vi "RealTimeSingleOld_NotInUse.vi"(4 "Frames/s":sgl=2.0, 5 "return to start":bool, 6 "Scan Axis":i8=3, 7 "Motion Board ID":T4=1 min=1 max=32 step=1, 8 "BKPT Shift":i32=75, 9 "stop":bool) -> (0 "error out":errorcluster, 2 "Bd ID Out":T3)   [LabVIEW 2022 SP3]
uses:
  ScanningControl/Motion Controllers/-MotionRoutines/MotionGlobals.vi
  <instrlib>/Acqiris Dx/Acqiris Dx.lvlib
  <vilib>/Motion/FlexMotion/FunctionsVIs/Trajectory.llb/Load Acceleration/Deceleration.flx
  <vilib>/Motion/FlexMotion/CustomControls/CustomControls.llb/Axis To Control.flx
  <vilib>/Motion/FlexMotion/CustomControls/CustomControls.llb/Program.flx
  <instrlib>/Newport ESP301/Newport ESP301.lvlib
  <instrlib>/niScope/Acquire/Fetch/niScope Multi Fetch Binary 8.vi
  ScanningControl/-ScanSystem/DataHandling/ReverseDataI8.vi
  <vilib>/DAQmx/write.llb/DAQmx Write (Digital 1D Bool NChan 1Samp 1Line).vi
  <instrlib>/LeCroy Wave Series/LeCroy Wave Series.lvlib
  <vilib>/Motion/FlexMotion/FunctionsVIs/Trajectory.llb/Wait for Move Complete (8 axes).flx
  <vilib>/Motion/FlexMotion/FunctionsVIs/StartStopMotion.llb/Start Motion (8 axes).flx
  <vilib>/Motion/FlexMotion/FunctionsVIs/StartStopMotion.llb/Stop Motion (8 axes).flx
panel:
  in  "Filter Prams":T1={"low cutoff"=20, "order"=81, "high cutoff"=60}
  in  "Type of Mean":u16(ring) items=["Mean from lines", "Mean just lines", "Poly Mean", "No mean", "Filter"]
  in  "Stop Motor":bool
  in  "Axis Tune":enum32{"Axis 1", "Axis 2", "Axis 3", "Axis 4"}(radio)=enum."Axis 2"
  in  "Position (mm) (Abs)":dbl format="%.3f"
  in  "Tabor":T2={"Time Step (ms)"=5000, "Burst Ct"=[1, 3, 5, 10, 20], "Voltage Steps"=[100.0], "Tabor Step Through?"=FALSE} {"Voltage Steps" format="%_3g"}
  in  "*.eye":bool
  in  "Movie Name":string="none"
  in  "BMP?":bool
  in  "view":bool=TRUE
  in  "distance?":bool=TRUE
  in  "Display mode":u16(ring)=1 items=["Linear Abs Grey", "Log Grey Scale", "Linear Color Scale", "Sector"]
  out "Raw data":dbl[][](graph)
  out "Frames":i32
  # "Cross Axis Motion"
  # "Set for 8 bit data"
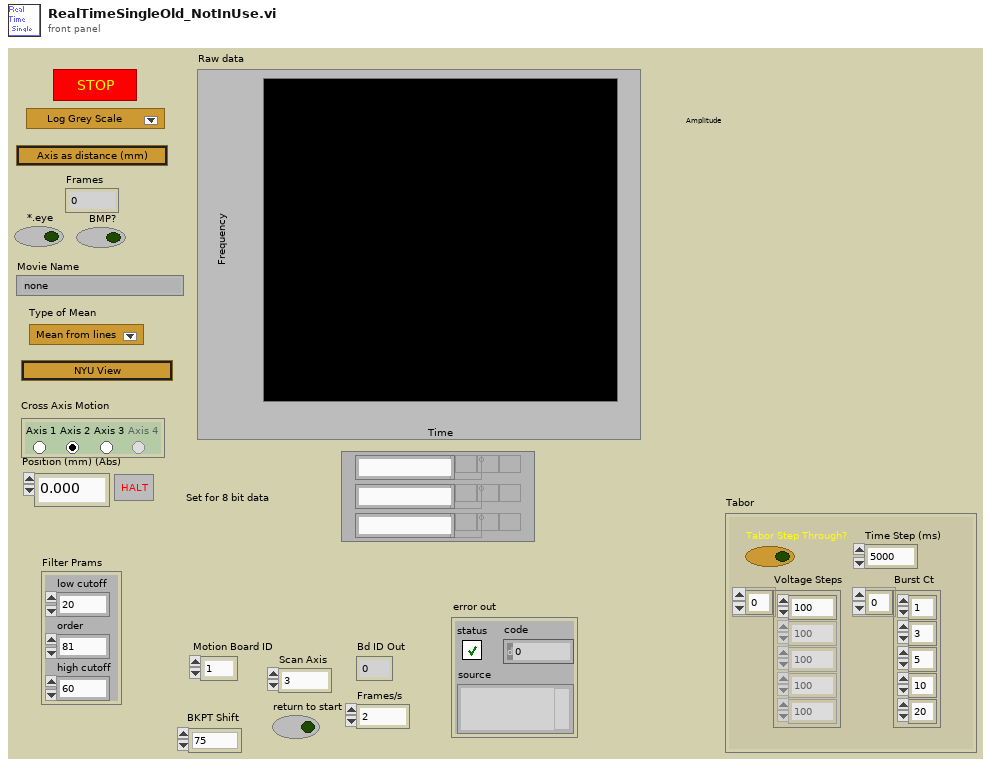
[diagram p1: front panel]
types:
  T1 = cluster{"low cutoff":i32, "order":i32, "high cutoff":i32}
  T2 = cluster{"Time Step (ms)":i64, "Burst Ct":i8[], "Voltage Steps":sgl[], "Tabor Step Through?":bool}
  T3 = typedef "Bd Id Out" = u8
  T4 = typedef "Board Id" = u8
  T5 = typedef "location.ctl" = enum16{"Automatic", "WCM Main", "Hawaii", "Columbia MM3000", "Columbia  NI System", "NYU", "RRI 2", "UHI Allen", "CUMC RT", "Chiba", "Stony Brook", "WCM Microscopy", "WCM Aeoretch", "WCM Optics Lab", "WCM Main 2Axis", "WCM Rotation", "WCM SAM SMAC", "SERI GP"}
  T6 = typedef "Program.flx" = u8
  T7 = cluster{"delay":sgl, "pivot distance":sgl, "sector scan angle":sgl, "operator":string, "Scan Mode":string, "location":string}
  T8 = cluster{"gain":dbl, bool, "Array":i16[][], "gain 2":dbl}
  T9 = typedef "Resource Out (Enum).flx" = u16
  T10 = typedef "Axis To Control.flx" = u16
  T11 = cluster{"X right":dbl, "X left":dbl, "Y low":dbl, "Y high":dbl}
  T12 = cluster{"Axis scaling Params":cluster{"X right":dbl, "X left":dbl, "Y low":dbl, "Y high":dbl}, "x scaled":dbl[][], "y scaled":dbl[][], "scales":cluster{"inc x (mm)":dbl, "inc y (mm)":dbl}, dbl[][]}
  T13 = cluster{"returnedSamplesPerSeg":i32, "indexFirstPoint":i32, "sampTime":dbl, "vGain":dbl, "vOffset":dbl, "returnedSegments":i32, "nbrAvgWforms":i32, "actualTriggersInAcqLo":u32, "actualTriggersInAcqHi":u32, "reserved3":dbl, "actualDataSize":u32, "missingValue":dbl}
  T14 = cluster{"actualSamples":i32, "absoluteInitialX":dbl, "relativeInitialX":dbl, "xIncrement":dbl, "offset":dbl, "gain":dbl, "reserved1":dbl, "reserved2":dbl}[]
  T15 = cluster{"actualSamples":i32, "absoluteInitialX":dbl, "relativeInitialX":dbl, "xIncrement":dbl, "offset":dbl, "gain":dbl, "reserved1":dbl, "reserved2":dbl}
  T16 = typedef "imagedata.ctl" = cluster{"image type":i32, "image depth":i32, "image":u8[], "mask":u8[], "colors":u32[], "Rectangle":cluster{"left":i16, "top":i16, "right":i16, "bottom":i16}}
  T17 = cluster{"gain":dbl, bool, "Array":i16[][], "gain 2 Ch":dbl}
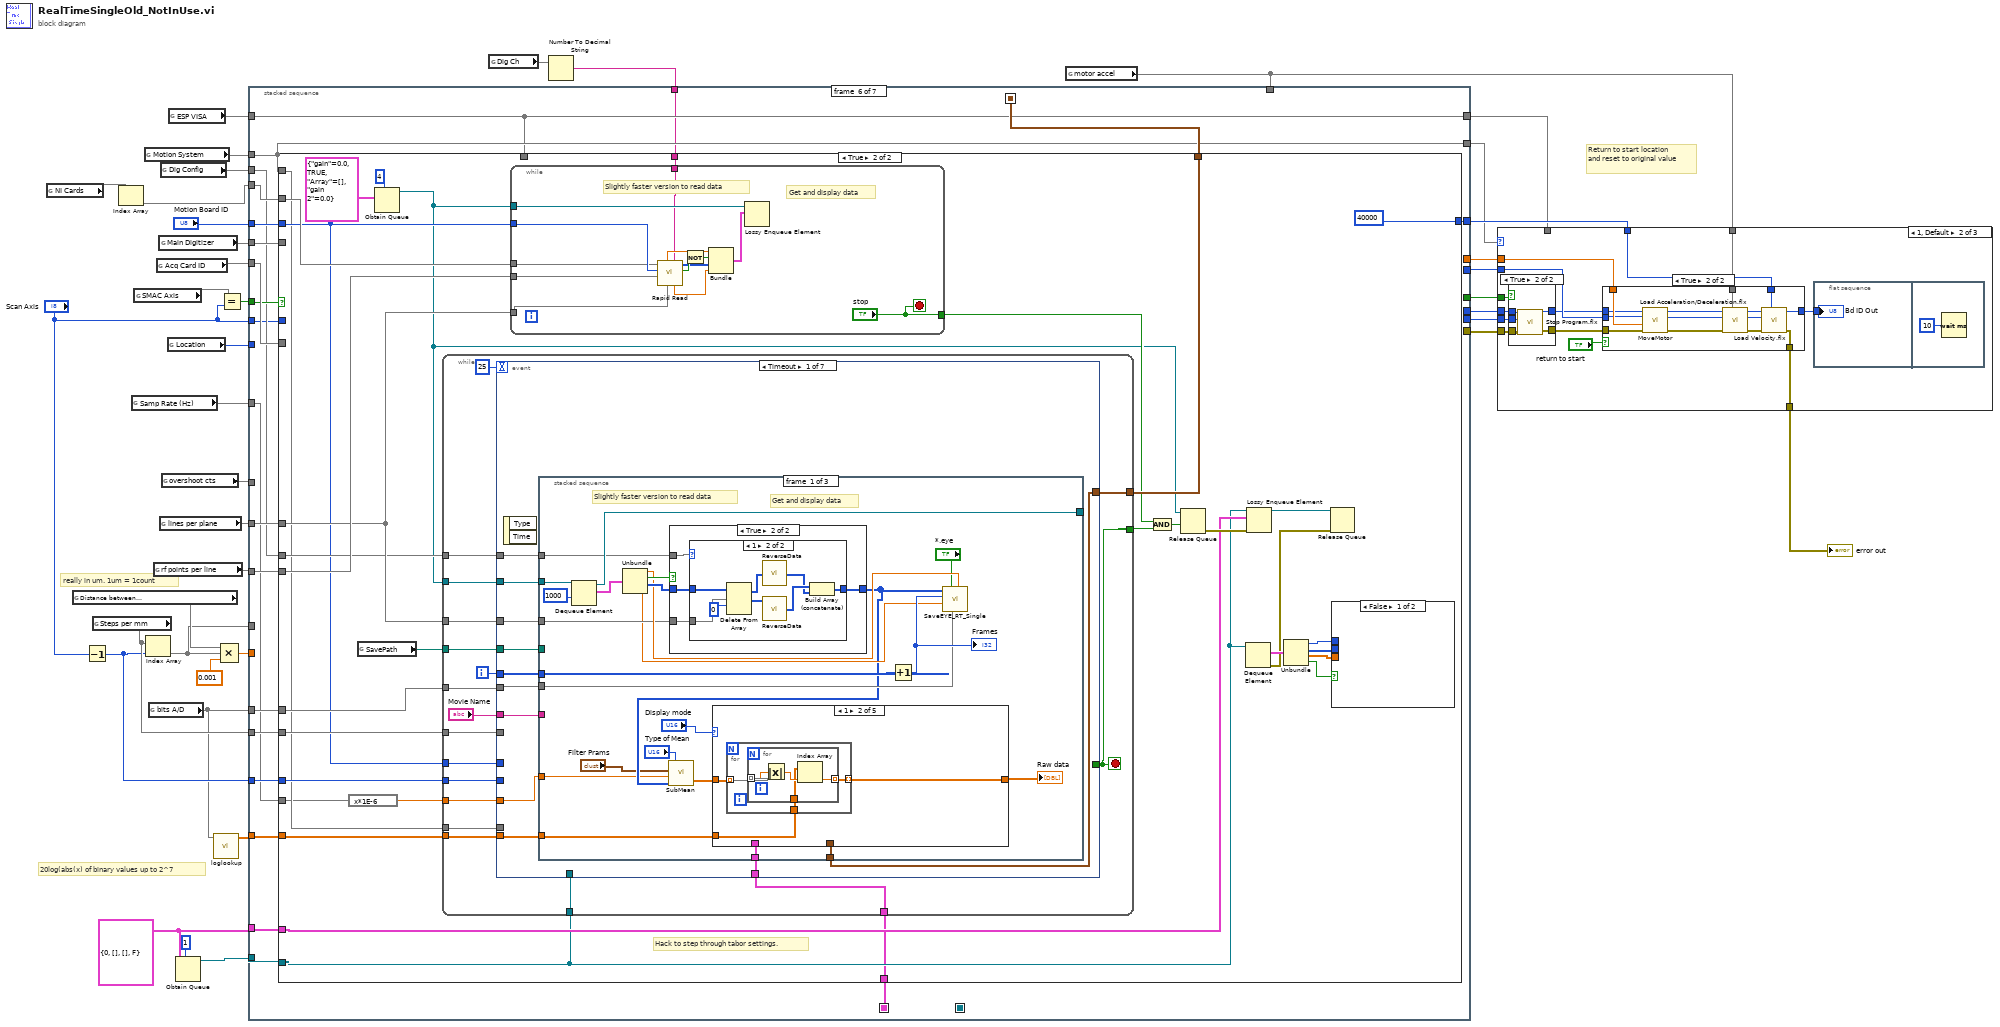
[diagram p0: block diagram]
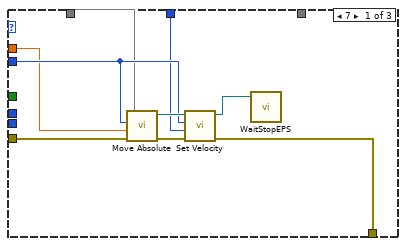
[diagram p2: hidden frame]
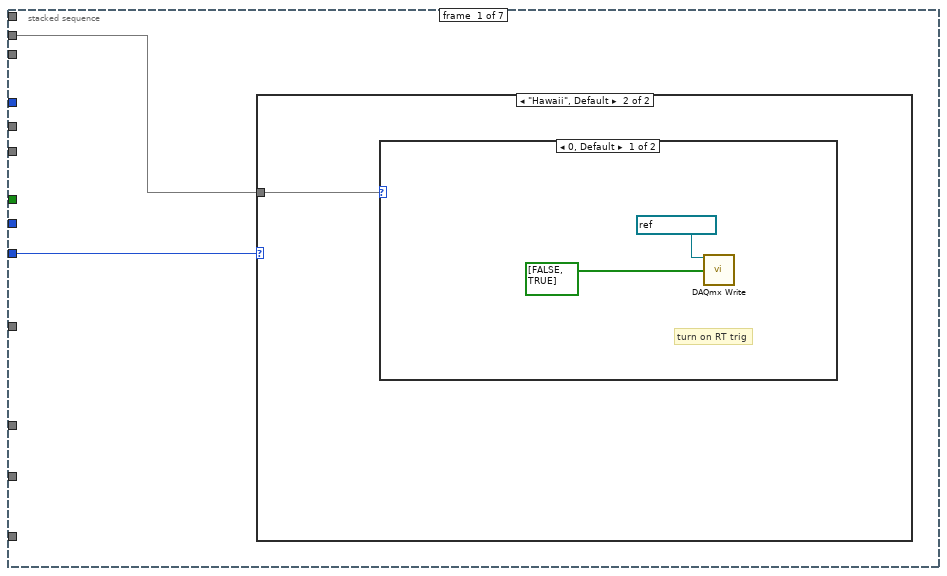
[diagram p6: hidden frame]
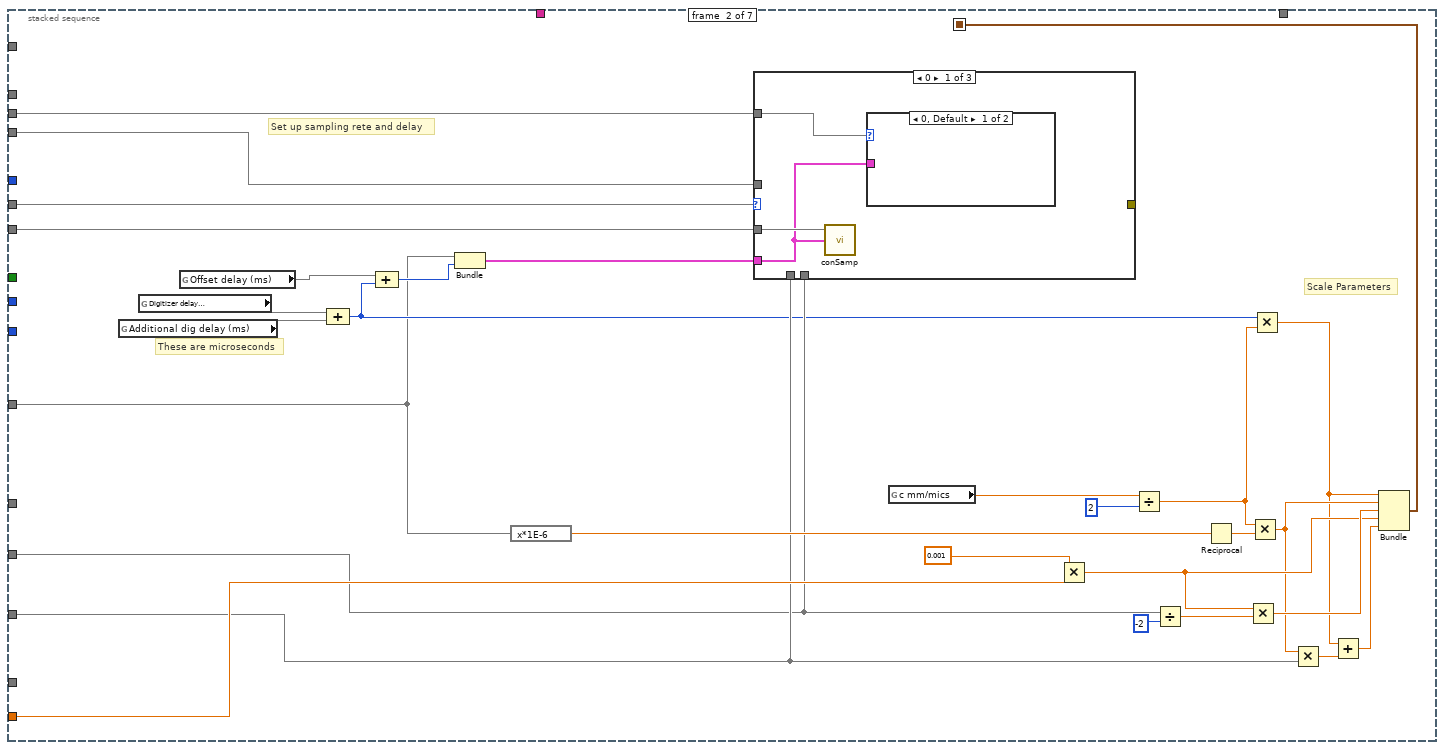
[diagram p9: hidden frame]
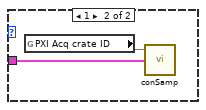
[diagram p10: hidden frame]
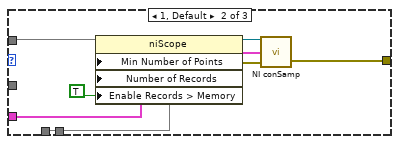
[diagram p11: hidden frame]
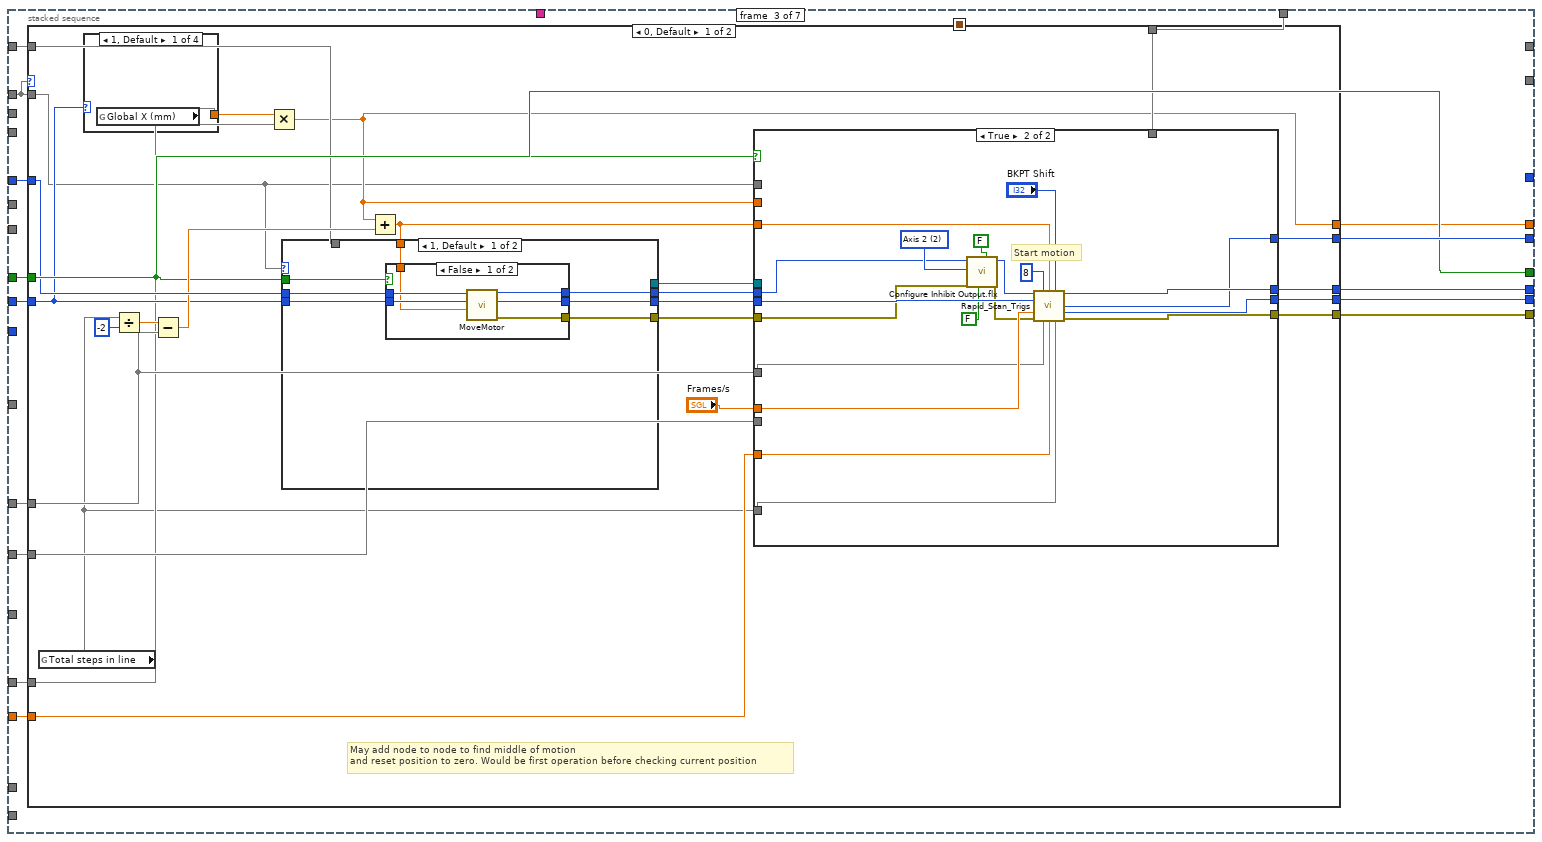
[diagram p13: hidden frame]
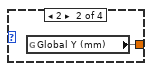
[diagram p14: hidden frame]
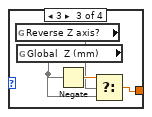
[diagram p15: hidden frame]
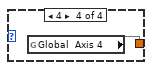
[diagram p16: hidden frame]
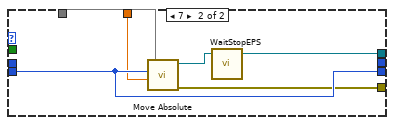
[diagram p18: hidden frame]
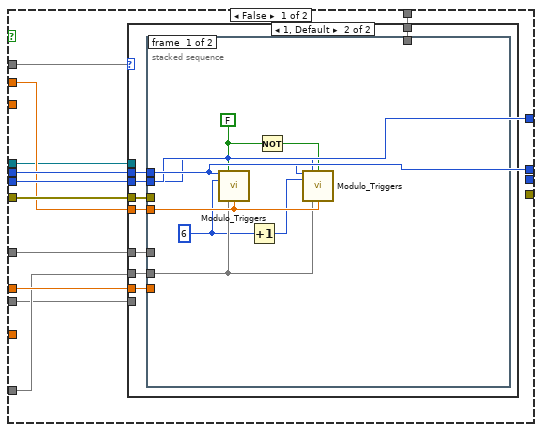
[diagram p19: hidden frame]
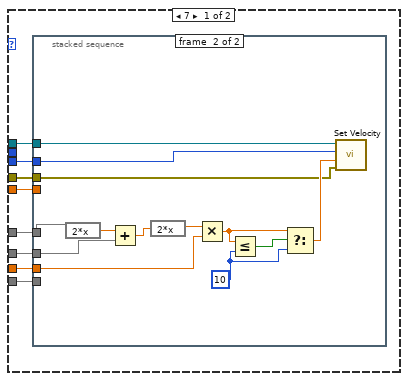
[diagram p20: hidden frame]
diagram:
  w8 = T2 {"Time Step (ms)"=0, "Burst Ct"=[], "Voltage Steps"=[], "Tabor Step Through?"=FALSE} ("Tabor")
  # "20log(abs(x) of binary values up to 2^7"
  # "really in um. 1um = 1count"
  # "Return to start location and reset to original value"
  n1 = global read "MotionGlobals.vi" "NI Cards"() -> (w11)
  n2 = global read "MotionGlobals.vi" "Distance between\nscan lines (mm)"() -> (w28)
  n3 = Decrement(x="Scan Axis") -> (x-1=w4:i8)
  n4 = global read "MotionGlobals.vi" "Steps per mm"() -> (w6)
  n5 = Index Array(array=w11) -> (element=w12)  [unwired: 1 in]
  n6 = global read "MotionGlobals.vi" "Samp Rate (Hz)"() -> (w3)
  n7 = global read "MotionGlobals.vi" "SMAC Axis"() -> (w10)
  n8 = global read "MotionGlobals.vi" "Motion System"() -> (w22)
  n9 = Index Array(array=w6, index=w4) -> (element=w13)
  n10 = global read "MotionGlobals.vi" "bits A/D"() -> (w2)
  n11 = global read "MotionGlobals.vi" "rf points per line"() -> (w39)
  n12 = global read "MotionGlobals.vi" "Acq Card ID"() -> (w25)
  n13 = global read "MotionGlobals.vi" "Main Digitizer"() -> (w26)
  n14 = global read "MotionGlobals.vi" "lines per plane"() -> (w40)
  n15 = global read "MotionGlobals.vi" "Dig Config"() -> (w16)
  n16 = global read "MotionGlobals.vi" "overshoot cts"() -> (w38)
  n17 = global read "MotionGlobals.vi" "Location"() -> (w17:T5)
  n18 = global read "MotionGlobals.vi" "ESP VISA"() -> (w21)
  n19 = Obtain Queue(max queue size (-1, unlimited)=1, element data type=w8) -> (queue out=w7:refnum<queue>)  [unwired: 3 in, 2 out]
  n20 = call "loglookup.vi"("A/D bits"=w2) -> ("Log Lookup"=w1:sgl[])  [unwired: 2 in, 2 out]
  n21 = Equal?(x=w10, y="Scan Axis") -> (x = y?=w30:bool)
  n22 = Compound Arithmetic op=MULTIPLY(w28, w13, 0.001) -> (w27:dbl)
  n23 = global read "MotionGlobals.vi" "Dig Ch"() -> (w15)
  n24 = Number To Decimal String(number=w15) -> (decimal integer string=w14:string)  [unwired: 1 in]
  n25 = global read "MotionGlobals.vi" "motor accel"() -> (w23)
  n26 = stacked-sequence {
    seq-local: [_ w63 _ _ _ _ _] -> [_ _ _ _ w298 w335 _]
    seq-local: [_ _ _ w260 _ _ _] -> [_ _ _ _ _ _ w772]
    seq-local: [_ _ _ _ w304 _ _] -> [_ _ _ _ _ w319 _]
    tunnel: w25 -> [_ w72 _ _ _ w339 _]
    tunnel: w40 -> [_ w51 w94 _ w303 w338 _]
    tunnel: [_ _ w102 _ _ _ _] -> w34
    tunnel: [_ _ w101 _ _ _ _] -> w36
    tunnel: w39 -> [_ w52 _ _ w302 w337 _]
    tunnel: [_ _ w100 _ _ _ _] -> w35
    tunnel: [_ _ w89 _ _ _ _] -> w33
    tunnel: w38 -> [_ _ w98 _ _ _ _]
    tunnel: [_ _ w99 _ _ _ _] -> w37
    tunnel: "Motion Board ID" -> [_ _ w97 w261 _ w336 _]
    tunnel: [_ _ w91 _ _ _ _] -> w31
    tunnel: w30 -> [_ _ w91 _ _ w334 _]
    tunnel: "Scan Axis" -> [_ _ w92 w262 _ w325 _]
    tunnel: w27 -> [_ w56 w96 _ _ _ _]
    tunnel: w26 -> [_ w55 _ _ _ w333 _]
    tunnel: w12 -> [_ w54 _ _ _ w332 _]
    tunnel: [_ _ _ _ _ w331 _] -> w24
    tunnel: w23 -> [_ _ w95 _ _ _ _]
    tunnel: w22 -> [_ _ w88 w264 _ w330 _]
    tunnel: w21 -> [_ _ w93 _ _ w329 _]
    tunnel: [_ _ _ _ _ w330 _] -> w20
    tunnel: [_ _ _ _ _ w329 _] -> w19
    tunnel: w17 -> [w42 _ _ _ _ _ w775]
    tunnel: w16 -> [w41 w47 _ w263 _ w328 w773]
    tunnel: w14 -> [_ _ _ _ _ w327 _]
    tunnel: w2 -> [_ _ _ _ _ w326 _]
    tunnel: w13 -> [_ _ w90 _ _ _ _]
    tunnel: w8 -> [_ _ _ _ _ w324 _]
    tunnel: w7 -> [_ _ _ _ _ w323 _]
    tunnel: w1 -> [_ _ _ _ _ w322 _]
    tunnel: w6 -> [_ _ _ _ _ w321 _]
    tunnel: w4 -> [_ _ _ w255 _ w320 _]
    tunnel: w3 -> [_ w46 _ _ w299 w318 _]
    frame #0 {
      n27 = case shown="\"Hawaii\", Default" w42 {
        tunnel: w41 -> [_ w43]
        frame "UHI Allen", "CUMC RT" {
        }
        frame "Hawaii", Default {
          n28 = case shown="0, Default" w43 {
            frame 0, Default {
              # "turn on RT trig"
              n29 = call-poly <vilib>:"DAQmx Write.vi"("task/channels in"=refnum<k21> "DIO-L2 L3", "data"=bool[] [FALSE, TRUE]) -> ()  [unwired: 11 in, 3 out]
            }
            frame 44 {
            }
          }
        }
      }
    }
    frame #1 {
      # "Scale Parameters"
      # "Set up sampling rete and delay"
      # "These are microseconds"
      n30 = global read "MotionGlobals.vi" "Additional dig delay (ms)"() -> (w74)
      n31 = global read "MotionGlobals.vi" "Digitizer delay\n (ms)"() -> (w70)
      n32 = global read "MotionGlobals.vi" "Offset delay (ms)"() -> (w50)
      n33 = Compound Arithmetic op=ADD(w70, w74) -> (w49:i32)
      n34 = Compound Arithmetic op=ADD(w50, w49) -> (w48:i32)
      n35 = Bundle("Samp Rate (Hz)"=w46, w48) -> (w73:cluster{"Samp Rate (Hz)":void, i32})  [unwired: 1 out]
      n36 = expression code="x*1E-6"(w46) -> (w53:dbl)
      n37 = case shown="0" w55 {
        tunnel: w73 -> [w76 w82 _]
        tunnel: w72 -> [w77 _ _]
        tunnel: w54 -> [_ w83 _]
        tunnel: w52 -> [_ w86 _]
        tunnel: w51 -> [_ w87 _]
        tunnel: [_ w81 _] -> _
        tunnel: w47 -> [w75 _ _]
        frame 0 {
          n38 = call "conSamp.vi"("Sampling"=w76, "InstrumentID"=w77) -> ()  [unwired: 1 in, 2 out]
          n39 = case shown="0, Default" w75 {
            tunnel: w76 -> [_ w79]
            frame 0, Default {
            }
            frame 1 {
              n40 = global read "MotionGlobals.vi" "PXI Acq crate ID"() -> (w78)
              n41 = call "conSamp.vi"("Sampling"=w79, "InstrumentID"=w78) -> ()  [unwired: 1 in, 2 out]
            }
          }
        }
        frame 1, Default {
          n42 = property class="niScope"(reference=w83, "Min Number of Points"=w86, "Number of Records"=w87, "Enable Records > Memory"=TRUE) -> (reference out=w85:refnum<k15>, error out=w84:errorcluster)  [unwired: 1 in]
          n43 = call "NI conSamp.vi"("error in"=w84, "Sampling"=w82, "InstrumentID"=w85) -> ("error out"=w81:errorcluster)  [unwired: 1 out]
        }
        frame 2 {
        }
      }
      n44 = global read "MotionGlobals.vi" "c mm/mics"() -> (w71:sgl)
      n45 = Multiply(x=0.001, y=w56) -> (x*y=w61:dbl)
      n46 = Divide(x=w71, y=2) -> (x/y=w64:sgl)
      n47 = Divide(x=w51, y=-2) -> (x/y=w66:dbl)
      n48 = Reciprocal(x=w53) -> (1/x=w69:dbl)
      n49 = Multiply(x=w61, y=w66) -> (x*y=w62:dbl)
      n50 = Multiply(x=w64, y=w69) -> (x*y=w60:dbl)
      n51 = Multiply(x=w49, y=w64) -> (x*y=w58:sgl)
      n52 = Multiply(x=w60, y=w52) -> (x*y=w59:dbl)
      n53 = Add(x=w58, y=w59) -> (x+y=w57:sgl)
      n54 = Bundle(w58, w60, w62, w61, w57) -> (w63:cluster{sgl, dbl, dbl, dbl, sgl})  [unwired: 1 out]
    }
    frame #2 {
      n55 = case shown="0, Default" w88 {
        tunnel: [w127 _] -> w102
        tunnel: [w126 _] -> w101
        tunnel: [w124 _] -> w100
        tunnel: [w123 _] -> w99
        tunnel: w98 -> [w121 _]
        tunnel: w97 -> [w117 _]
        tunnel: w96 -> [w116 _]
        tunnel: w95 -> [w114 _]
        tunnel: w94 -> [w113 _]
        tunnel: w93 -> [w112 _]
        tunnel: w92 -> [w110 _]
        tunnel: w91 -> [w108 _]
        tunnel: w90 -> [w106 _]
        tunnel: [w105 _] -> w89
        tunnel: w88 -> [w104 _]
        frame 0, Default {
          # "May add node to node to find middle of motion\nand reset position to zero. Would be first operation before checking current position"
          n56 = global read "MotionGlobals.vi" "Total steps in line"() -> (w103)
          n57 = case shown="1, Default" w110 {
            tunnel: [w129 w130 w131 w135] -> w107
            frame 1, Default {
              n58 = global read "MotionGlobals.vi" "Global X (mm)"() -> (w129)
            }
            frame 2 {
              n59 = global read "MotionGlobals.vi" "Global Y (mm)"() -> (w130)
            }
            frame 3 {
              n60 = global read "MotionGlobals.vi" "Reverse Z axis?"() -> (w132)
              n61 = global read "MotionGlobals.vi" "Global  Z (mm)"() -> (w133)
              n62 = Negate(x=w133) -> (-x=w134:dbl)
              n63 = Select(t=w134, s=w132, f=w133) -> (s? t:f=w131:dbl)
            }
            frame 4 {
              n64 = global read "MotionGlobals.vi" "Global  Axis 4"() -> (w135)
            }
          }
          n65 = Divide(x=w103, y=-2) -> (x/y=w122:dbl)
          n66 = Subtract(x=w122, y=w121) -> (x-y=w115:dbl)
          n67 = Multiply(x=w107, y=w106) -> (x*y=w105:dbl)
          n68 = Add(x=w105, y=w115) -> (x+y=w109:dbl)
          n69 = case shown="1, Default" w104 {
            tunnel: [w140 _] -> w120
            tunnel: [w139 w156] -> w119
            tunnel: [w138 w153] -> w118
            tunnel: w117 -> [w142 _]
            tunnel: w110 -> [w141 w156]
            tunnel: w112 -> [_ w152]
            tunnel: [_ w154] -> w111
            tunnel: w109 -> [w137 w151]
            tunnel: w108 -> [w136 _]
            frame 1, Default {
              n70 = case shown="False" w136 {
                tunnel: w142 -> [w148 w150]
                tunnel: w141 -> [w147 w149]
                tunnel: [w146 w150] -> w140
                tunnel: [w145 w149] -> w139
                tunnel: [w144 _] -> w138
                tunnel: w137 -> [w143 _]
                frame False {
                  n71 = call "MoveMotor.vi"("Target Position (0)"=w143, "Axis or Vector Space"=w147, "Motion Bd ID"=w148) -> ("error out"=w144:errorcluster, "Resource Output"=w145:u16, "Bd ID Out"=w146:u8)  [unwired: 2 in, 4 out]
                }
                frame True {
                }
              }
            }
            frame 7 {
              n72 = call <instrlib>:"Move Absolute.vi"("Position (0 units)"=w151, "Axis (1)"=w156, "VISA resource name"=w152) -> ("error out"=w153:errorcluster, "VISA resource name out"=w155:refnum<visa-resource-name>)  [unwired: 3 in]
              n73 = call "WaitStopEPS.vi"("VISA resource name"=w155) -> ("VISA resource name out"=w154:refnum<visa-resource-name>)  [unwired: 2 in, 2 out]
            }
          }
          n74 = case shown="True" w108 {
            tunnel: "Frames/s" -> [w164 w253]
            tunnel: [_ w252] -> w127
            tunnel: [w167 w251] -> w126
            tunnel: [_ w250] -> w124
            tunnel: [w166 w249] -> w123
            tunnel: w103 -> [w160 w248]
            tunnel: w116 -> [_ w247]
            tunnel: w121 -> [w165 w246]
            tunnel: w120 -> [w167 w236]
            tunnel: w119 -> [w166 w245]
            tunnel: w118 -> [w163 w235]
            tunnel: w109 -> [_ w244]
            tunnel: w105 -> [w162 _]
            tunnel: w114 -> [w161 _]
            tunnel: w113 -> [w159 _]
            tunnel: w104 -> [w158 _]
            tunnel: w111 -> [w157 _]
            frame False {
              n75 = case shown="1, Default" w158 {
                tunnel: w160 -> [w175 w209]
                tunnel: w167 -> [_ w208]
                tunnel: w166 -> [w170 w207]
                tunnel: w165 -> [w172 w206]
                tunnel: w164 -> [w171 w205]
                tunnel: w163 -> [w168 w204]
                tunnel: w162 -> [w173 w203]
                tunnel: w161 -> [_ w202]
                tunnel: w159 -> [w174 _]
                tunnel: w157 -> [w169 _]
                frame 7 {
                  n76 = stacked-sequence {
                    tunnel: w175 -> [w180 w194]
                    tunnel: w174 -> [w177 _]
                    tunnel: w173 -> [w179 _]
                    tunnel: w172 -> [_ w195]
                    tunnel: w171 -> [_ w193]
                    tunnel: w170 -> [w178 w191]
                    tunnel: w169 -> [w188 w190]
                    tunnel: w168 -> [w183 w189]
                    frame #0 {
                      n77 = call "ESP_Upload_Long.vi"("Motion Settings In"=w188, "Axis"=w178, "Purge?"=TRUE, "lines per scan"=w177, "Program#"=1, "Reverse ?"=FALSE, "error in"=w183, 12:w180, "Offset"=w179) -> ("VISA resource name out"=w187:refnum<visa-resource-name>, "error out"=w182:errorcluster)  [unwired: 5 in]
                      n78 = call "ESP_Upload_Long.vi"("Motion Settings In"=w187, "Axis"=w178, "lines per scan"=w177, "Program#"=2, "Reverse ?"=TRUE, "error in"=w182, 12:w180, "Offset"=w179) -> ()  [unwired: 6 in, 2 out]
                    }
                    frame #1 {
                      w200 = 10
                      n79 = expression code="2*x"(w195) -> (w198:dbl)
                      n80 = Add(x=w198, y=w194) -> (x+y=w196:dbl)
                      n81 = expression code="2*x"(w196) -> (w197:dbl)
                      n82 = Multiply(x=w197, y=w193) -> (x*y=w201:sgl)
                      n83 = Less Or Equal?(x=w201, y=w200) -> (x <= y?=w199:bool)
                      n84 = Select(t=w201, s=w199, f=w200) -> (s? t:f=w192:sgl)
                      n85 = call <instrlib>:"Set Velocity.vi"("error in (no error)"=w189, "Velocity (units/s)"=w192, "Axis (1)"=w191, "VISA resource name"=w190) -> ()  [unwired: 2 in, 2 out]
                    }
                  }
                }
                frame 1, Default {
                  n86 = stacked-sequence {
                    tunnel: w203 -> [w217 _]
                    tunnel: w209 -> [w216 w231]
                    tunnel: w208 -> [w212 w227]
                    tunnel: w207 -> [w211 w226]
                    tunnel: w206 -> [_ w224]
                    tunnel: w205 -> [_ w222]
                    tunnel: w204 -> [_ w228]
                    tunnel: w202 -> [_ w218]
                    frame #0 {
                      w210 = T6 6 ("Program (1)")
                      w215 = FALSE
                      n87 = call "Modulo_Triggers.vi"("Motion Settings In"=w212, "Axis"=w211, "Reverse ?"=w215, "Program (1)"=w210, 12:w216, "Offset"=w217) -> ()  [unwired: 2 in, 8 out]
                      n88 = Increment(x=w210) -> (x+1=w213:T6)
                      n89 = Not(x=w215) -> (.not. x?=w214:bool)
                      n90 = call "Modulo_Triggers.vi"("Motion Settings In"=w212, "Axis"=w211, "Reverse ?"=w214, "Program (1)"=w213, 12:w216, "Offset"=w217) -> ()  [unwired: 2 in, 8 out]
                    }
                    frame #1 {
                      w233 = 100000
                      n91 = expression code="2*x"(w224) -> (w223:dbl)
                      n92 = Add(x=w223, y=w231) -> (x+y=w220:dbl)
                      n93 = expression code="2*x"(w220) -> (w221:dbl)
                      n94 = Multiply(x=w221, y=w222) -> (x*y=w234:sgl)
                      n95 = Less Or Equal?(x=w234, y=w233) -> (x <= y?=w232:bool)
                      n96 = Select(t=w234, s=w232, f=w233) -> (s? t:f=w219:sgl)
                      n97 = call <vilib>:"Load Velocity.flx"("Velocity (10000)"=w219, "error in (no error)"=w228, "Axis or Vector Space"=w226, "Board ID"=w227) -> ("error out"=w229:errorcluster, "Resource Output"=w225:T9, "Bd ID Out"=w230:T3)  [unwired: 3 out]
                      n98 = call "Load Acceleration/Deceleration.flx"("Acceleration (100000)"=w218, "error in (no error)"=w229, "Axis or Vector Space"=w225, "Board ID"=w230) -> ()  [unwired: 1 in, 5 out]
                    }
                  }
                }
              }
            }
            frame True {
              w239 = T10 2 items=["Axis 1"=1, "Axis 2"=2, "Axis 3"=3, "Axis 4"=4, "Axis 5"=5, "Axis 6"=6, "Axis 7"=7, "Axis 8"=8] ("Axis")
              # "Start motion"
              n99 = call <vilib>:"Configure Inhibit Output.flx"("Enable"=FALSE, "Polarity (Active Low)"=FALSE, "error in (no error)"=w235, "Axis"=w239, "Board ID"=w236) -> ("error out"=w242:errorcluster, "Bd ID Out"=w243:T3)  [unwired: 1 in, 4 out]
              n100 = call "Rapid_Scan_Trigs.vi"("Board ID"=w243, "Program (1)"=T6 8, "Start Position"=w244, "BKPT Shift"="BKPT Shift", "Scan Axis"=w245, "# frames/ s"=w253, "error in (no error)"=w242, "overshoot"=w246, "step interval"=w247, "Total Steps (one way)"=w248) -> ("Bd ID Out"=w251:u8, "Axis Resource out"=w249:u16, "Program ID"=w250:u8, "error out"=w252:errorcluster)  [unwired: 1 in, 1 out]
            }
          }
        }
        frame 8 {
        }
      }
    }
    frame #3 {
      # "Lock out axis of SMAC and update position"
      n101 = case shown="0, Default" w263 {
        tunnel: [_ w280] -> w260
        tunnel: w262 -> [_ w283]
        tunnel: w261 -> [_ w276]
        frame 0, Default {
        }
        frame 4 {
          n102 = global read "MotionGlobals.vi" "Switch T/R"() -> (w275)
          n103 = Decrement(x=w275) -> (x-1=w274:dbl)
          n104 = Replace Array Subset(array=bool[] [FALSE, FALSE, FALSE, FALSE, FALSE] ("XMIT"), new element=TRUE ("new element/subarray"), index=w274) -> (w271:bool[])
          n105 = call "5ChPulserTrigsNew.vi"("Motion Settings"=w276, "XMIT"=w271, "Axis"=w283) -> ("5CH Pulser Tasks"=w282:refnum<k21>[])  [unwired: 6 in, 1 out]
          n106 = for {
            tunnel: w282 -> [w295] mode=indexing
            tunnel: [w294] -> w280 mode=indexing
            tunnel: [w293] -> w279
            n107 = call <vilib>:"DAQmx Start Task.vi"("task/channels in"=w295) -> ("task out"=w294:refnum<k21>, "error out"=w293:errorcluster)  [unwired: 1 in, 12 out]
          }
          n108 = for {
            tunnel: bool[][] [[TRUE], [FALSE]] ("data") -> [w287] mode=indexing
            tunnel: w279 -> [_]
            tunnel: [w286] -> w277
            n109 = flat-sequence {
              tunnel: w287 -> [w290]
              tunnel: [w290] -> w288
              tunnel: w288 -> [w292]
              tunnel: [w291] -> w286
              frame #0 {
                n110 = Wait (ms)(milliseconds to wait=u32 25) -> ()  [unwired: 1 out]
              }
              frame #1 {
                n111 = call "DAQ Assistant"("data"=w292) -> ("error out"=w291:errorcluster)  [unwired: 17 in, 1 out]
              }
            }
          }
          n112 = for {
            N: 3 -> [_]
            tunnel: w276 -> [w285]
            tunnel: w277 -> [w284]
            n113 = call "ForceBreakPt.vi"("error in"=w284, "Bd ID in"=w285) -> ()  [unwired: 2 out]
          }
        }
      }
      n114 = Replace Array Subset(array=i32[] [0, 0, 0, 0], new element=2 ("new element/subarray"), index=w255) -> (w258:i32[])
      n115 = local read "Axis Tune"() -> (w259:enum32{"Axis 1", "Axis 2", "Axis 3", "Axis 4"})
      n116 = local read "distance?"() -> (w254:bool)
      n117 = case shown="0, Default" w264 {
        tunnel: w261 -> [w296 _]
        frame 0, Default {
          n118 = call "CheckLimStat.vi"("Motion Board ID"=w296) -> ()
        }
        frame 1, 7, 8 {
        }
      }
      n119 = for {
        tunnel: w258 -> [w265] mode=indexing
        i -> [w266]
        n120 = case shown="3" w266 {
          tunnel: w265 -> [w267 w268 w269 w270]
          frame 0, Default {
            n121 = property on="Axis 1" class="Bool (strict)"("DisabledEnum"=w267) -> ()  [unwired: 2 in, 2 out]
          }
          frame 1 {
            n122 = property on="Axis 2" class="Bool (strict)"("DisabledEnum"=w268) -> ()  [unwired: 2 in, 2 out]
          }
          frame 2 {
            n123 = property on="Axis 3" class="Bool (strict)"("DisabledEnum"=w269) -> ()  [unwired: 2 in, 2 out]
          }
          frame 3 {
            n124 = property on="Axis 4" class="Bool (strict)"("DisabledEnum"=w270) -> ()  [unwired: 2 in, 2 out]
          }
        }
      }
      n125 = property on="Axis Tune" class="RadioBtnsControl (strict)"("Val(Sgnl)"=w259) -> ()  [unwired: 2 in, 2 out]
      n126 = property on="distance?" class="Bool (strict)"("Val(Sgnl)"=w254) -> ()  [unwired: 2 in, 2 out]
    }
    frame #4 {
      w305 = i16 1000  # pixels in y
      w306 = i16 256  # pixels in x
      # "Precalc for sector images"
      n127 = Build Array(w303, w302) -> (w301:void[])
      n128 = Unbundle(w298) -> (w297:sgl)  [unwired: 4 out]
      n129 = Bundle By Name(cluster=T7 {"delay"=0.0, "pivot distance"=0.0, "sector scan angle"=0.0, "operator"="", "Scan Mode"="", "location"=""} ("Scan Info"), "delay"=w297, "pivot distance"=sgl 9.0, "sector scan angle"=sgl 50.0) -> (w310:T7)
      n130 = expression code="x*1E-6"(w299) -> (w300:dbl)
      n131 = Reciprocal(x=w300) -> (1/x=w314:dbl)
      n132 = call "SecOverlayParams.vi"("Scan Info"=w310, "Time between rf pts\nmicros"=w314, "pixels in y"=w305, "Array"=w301, "pixels in x"=w306) -> ("scales"=w309:cluster{"inc x (mm)":dbl, "inc y (mm)":dbl}, "y scaled"=w315:dbl[][], "x scaled"=w316:dbl[][], "Axis scaling Params"=w317:T11)  [unwired: 3 in]
      n133 = Initialize Array(0.0 ("element"), w306, w305) -> (w307:dbl[][])
      n134 = Bundle("Axis scaling Params"=w317, "x scaled"=w316, "y scaled"=w315, "scales"=w309, w307) -> (w304:T12)  [unwired: 1 in]
    }
    frame #5 {
      n135 = case shown="True" w334 {
        tunnel: w339 -> [w354 _]
        tunnel: w338 -> [w355 w534]
        tunnel: w337 -> [w356 w550]
        tunnel: w336 -> [w352 w523]
        tunnel: w335 -> [w351 w548]
        tunnel: w333 -> [w350 _]
        tunnel: w332 -> [w349 w542]
        tunnel: [w348 40000] -> w331
        tunnel: w330 -> [w347 w522]
        tunnel: w329 -> [w346 _]
        tunnel: w328 -> [_ w533]
        tunnel: w327 -> [w345 w531]
        tunnel: w326 -> [w344 w530]
        tunnel: w325 -> [w342 _]
        tunnel: w324 -> [_ w529]
        tunnel: w323 -> [w341 w528]
        tunnel: w322 -> [_ w526]
        tunnel: w321 -> [_ w525]
        tunnel: w320 -> [_ w524]
        tunnel: w319 -> [_ w520]
        tunnel: w318 -> [_ w519]
        frame False {
          n136 = global read "MotionGlobals.vi" "DigTimeOut"() -> (w343)
          n137 = while {
            tunnel: w356 -> [w385]
            tunnel: w355 -> [w375]
            tunnel: w354 -> [w384]
            shift-right: [w383] -> _
            shift-left: TRUE -> [w367]
            tunnel: w352 -> [w382]
            tunnel: w351 -> [w378]
            tunnel: w350 -> [w376]
            tunnel: w349 -> [w374]
            tunnel: w347 -> [w368]
            tunnel: w346 -> [w369]
            tunnel: w345 -> [w362]
            tunnel: w344 -> [w360]
            tunnel: w343 -> [w359]
            tunnel: w342 -> [w358]
            tunnel: w341 -> [w357]
            tunnel: [w357] -> w340
            i -> [w377]
            stop <- w381 stop-if-true
            # "Display data"
            # "Get data"
            # "This is slower version for heavier mass motors. Scan stop, read data, scan etc"
            n138 = Select(t="1", s=w367, f="2") -> (s? t:f=w364:string)
            n139 = Select(t=T6 6 ("Program (1)"), s=w367, f=T6 7 ("Program (1)")) -> (s? t:f=w372:T6)
            n140 = case shown="2" w376 {
              tunnel: w385 -> [w402 w445 _]
              tunnel: w375 -> [w401 w440 w479]
              tunnel: w384 -> [w415 _ _]
              tunnel: w382 -> [w414 w459 w468]
              tunnel: [w413 w458 w493] -> w380
              tunnel: w372 -> [w409 w457 w492]
              tunnel: [w395 w450 w474] -> w361
              tunnel: w374 -> [_ w451 _]
              tunnel: w367 -> [w398 w447 w473]
              tunnel: [w399 w448 w475] -> w373
              tunnel: w368 -> [w393 _ w487]
              tunnel: w369 -> [w397 _ w490]
              tunnel: w364 -> [w396 _ w489]
              tunnel: [w391 w437 w472] -> w363
              tunnel: w362 -> [_ w446 _]
              tunnel: w359 -> [w390 w434 w477]
              tunnel: w358 -> [_ _ w467]
              frame 0 {
                n141 = call <instrlib>:"Configure Memory Settings.vi"("Number of Samples (1000)"=w402, "Number of Segments (1)"=w401, "Instrument ID"=w415) -> ("error out"=w412:errorcluster, "dup Instrument ID"=w410:u32)  [unwired: 1 in, 2 out]
                n142 = call <instrlib>:"Start Acquisition.vi"("error in (no error)"=w412, "Instrument ID"=w410) -> ("error out"=w408:errorcluster, "dup Instrument ID"=w411:u32)  [unwired: 2 in]
                n143 = stacked-sequence {
                  tunnel: w408 -> [w433]
                  tunnel: [w433] -> w407
                  frame #0 {
                    n144 = Wait (ms)(milliseconds to wait=20) -> ()  [unwired: 1 out]
                  }
                }
                n145 = case shown="7" w393 {
                  tunnel: w414 -> [w421 _]
                  tunnel: [w420 _] -> w413
                  tunnel: w409 -> [w419 _]
                  tunnel: w407 -> [w418 w426]
                  tunnel: [w417 w423] -> w406
                  tunnel: w397 -> [_ w425]
                  tunnel: w396 -> [_ w424]
                  tunnel: [_ w422] -> w394
                  frame 0, Default {
                    n146 = call <vilib>:"Run Program.flx"("error in (no error)"=w418, "Program (1)"=w419, "Board ID"=w421) -> ("error out"=w417:errorcluster, "Bd ID Out"=w420:T3)  [unwired: 4 out]
                  }
                  frame 7 {
                    n147 = call <instrlib>:"Execute Program.vi"("error in (no error)"=w426, "Program Name"=w424, "VISA resource name"=w425) -> ("error out"=w423:errorcluster, "VISA resource name out"=w422:refnum<visa-resource-name>)  [unwired: 3 in]
                  }
                }
                n148 = expression code="x*1000"(w390) -> (w389:dbl)
                n149 = stacked-sequence {
                  tunnel: w406 -> [w430]
                  tunnel: [w430] -> w405
                  frame #0 {
                    n150 = Wait (ms)(milliseconds to wait=20) -> ()  [unwired: 1 out]
                  }
                }
                n151 = call "WaitForSegs.vi"("Acqiris ID"=w411, "lines per plane"=w401, "error in"=w405, "Timeout"=w389) -> ("dup Instrument ID"=w404:u32, "error out"=w403:errorcluster)  [unwired: 2 out]
                n152 = call "GetWaveform.vi"("Acq ID Out"=w404, "Num Samps"=w402, "Num Segs"=w401, "error in"=w403) -> ("Acquired Waveform16 bit"=w400:i16[][], "dataDesc"=w392:T13, "error out"=w395:errorcluster)  [unwired: 2 in, 7 out]
                n153 = case shown="True" w398 {
                  tunnel: w400 -> [w427 w429]
                  tunnel: [w427 w428] -> w399
                  frame False {
                  }
                  frame True {
                    n154 = call "ReverseData.vi"("Array in"=w429) -> ("Array out"=w428:i16[][])
                  }
                }
                n155 = Unbundle By Name(w392) -> ("vGain"=w391:dbl)
                n156 = case shown="7" w393 {
                  tunnel: w394 -> [_ w416]
                  frame 0, Default {
                  }
                  frame 7 {
                    n157 = call "WaitStopEPS.vi"("VISA resource name"=w416) -> ()  [unwired: 2 in, 3 out]
                  }
                }
              }
              frame 1, Default {
                n158 = property class="niScope"(reference=w451, "Number of Records"=w440, "Min Number of Points"=w445) -> (reference out=w453:refnum<k15>, error out=w452:errorcluster)  [unwired: 1 in]
                n159 = call <instrlib>:"niScope Initiate Acquisition.vi"("instrument handle"=w453, "error in"=w452) -> ("instrument handle out"=w444:refnum<k15>, "error out"=w456:errorcluster)  [unwired: 1 in, 11 out]
                n160 = stacked-sequence {
                  tunnel: w456 -> [w466]
                  tunnel: [w466] -> w455
                  frame #0 {
                    n161 = Wait (ms)(milliseconds to wait=u32 5) -> ()  [unwired: 1 out]
                  }
                }
                n162 = call <vilib>:"Run Program.flx"("error in (no error)"=w455, "Program (1)"=w457, "Board ID"=w459) -> ("error out"=w454:errorcluster, "Bd ID Out"=w458:T3)  [unwired: 4 out]
                n163 = stacked-sequence {
                  tunnel: w454 -> [w463]
                  tunnel: [w463] -> w442
                  frame #0 {
                    n164 = Wait (ms)(milliseconds to wait=u32 20) -> ()  [unwired: 1 out]
                  }
                }
                n165 = property class="niScope"(reference=w444, error in=w442, "Fetch Record Number"=0, "Fetch Number of Records"=-1) -> (reference out=w443:refnum<k15>, error out=w441:errorcluster)
                n166 = call-poly <instrlib>:"niScope Fetch (poly).vi"("timeout"=w434, "error in"=w441, "numSamples"=w445, "channels"=w446, "instrument handle"=w443) -> ("error out"=w450:errorcluster, "wfm"=w449:i8[][], "wfm info"=w439:T14)  [unwired: 4 out]
                n167 = case shown="True" w447 {
                  tunnel: w449 -> [w460 w462]
                  tunnel: [w460 w461] -> w448
                  frame False {
                  }
                  frame True {
                    n168 = call-poly "ReversePoly.vi"("Array in"=w462) -> ("Array out"=w461:i8[][])
                  }
                }
                n169 = Index Array(array=w439) -> (element=w438:T15)  [unwired: 1 in]
                n170 = Unbundle By Name(w438) -> ("gain"=w437:dbl)
              }
              frame 2 {
                w486 = FALSE ("Continuous Acquisition Mode (T: On)")
                w484 = u16 2 items=["RealTime", "RIS", "Sequence", "Roll", "WaveStream"] ("Sample Mode (0: RealTime)")
                n171 = global read "MotionGlobals.vi" "LeCroy"() -> (w478)
                n172 = call <instrlib>:"Configure Continuous Acquisition.vi"("Auto Trigger Enabled (T: Normal)"=w486, "Continuous Acquisition Mode (T: On)"=w486, "VISA resource name"=w478) -> ("error out"=w483:errorcluster, "VISA resource name out"=w485:refnum<visa-resource-name>)  [unwired: 7 in]
                n173 = call <instrlib>:"Configure Sample Mode.vi"("error in (no error)"=w483, "Number of Segments (2)"=w479, "Sample Mode (0: RealTime)"=w484, "VISA resource name"=w485) -> ("error out"=w482:errorcluster, "VISA resource name out"=w480:refnum<visa-resource-name>)  [unwired: 6 in]
                n174 = call <instrlib>:"Initiate.vi"("error in (no error)"=w482, "VISA resource name"=w480) -> ("error out"=w481:errorcluster)  [unwired: 8 in, 1 out]
                n175 = case shown="0, Default" w487 {
                  tunnel: w468 -> [w499 _]
                  tunnel: [w498 _] -> w493
                  tunnel: w492 -> [w497 _]
                  tunnel: w481 -> [w496 w504]
                  tunnel: [w495 w501] -> w491
                  tunnel: w490 -> [_ w503]
                  tunnel: w489 -> [_ w502]
                  tunnel: [_ w500] -> w488
                  frame 0, Default {
                    n176 = call <vilib>:"Run Program.flx"("error in (no error)"=w496, "Program (1)"=w497, "Board ID"=w499) -> ("error out"=w495:errorcluster, "Bd ID Out"=w498:T3)  [unwired: 4 out]
                  }
                  frame 7 {
                    n177 = call <instrlib>:"Execute Program.vi"("error in (no error)"=w504, "Program Name"=w502, "VISA resource name"=w503) -> ("error out"=w501:errorcluster, "VISA resource name out"=w500:refnum<visa-resource-name>)  [unwired: 3 in]
                  }
                }
                n178 = expression code="x*1000"(w477) -> (w469:dbl)
                n179 = stacked-sequence {
                  tunnel: w491 -> [w505]
                  tunnel: [w505] -> w470
                  frame #0 {
                    n180 = Wait (ms)(milliseconds to wait=40) -> ()  [unwired: 1 out]
                  }
                }
                n181 = call-poly <vilib>:"Wait for Move Complete.flx"("Timeout (10000 ms)"=w469, "error in (no error)"=w470, "Axis or Vector Space"=w467, "Board ID"=w468) -> ("error out"=w471:errorcluster)  [unwired: 4 in, 3 out]
                n182 = call "GetAcqSeqLeCroy.vi"("errorin"=w471, "save?"=FALSE, "Reverse?"=w473) -> ("Raw VGain (scale)"=w472:dbl, "Data Array"=w475:i16[][], "error out"=w474:errorcluster)  [unwired: 18 in, 4 out]
                n183 = case shown="7" w487 {
                  tunnel: w488 -> [_ w494]
                  frame 0, Default {
                  }
                  frame 7 {
                    n184 = call "WaitStopEPS.vi"("VISA resource name"=w494) -> ()  [unwired: 2 in, 3 out]
                  }
                }
              }
            }
            n185 = case shown="No Error" w361 {
              selector: w361 -> [w511 w516]
              tunnel: [w512 w516] -> w379
              tunnel: [w515 TRUE] -> w381
              tunnel: w378 -> [w514 _]
              tunnel: w377 -> [w513 _]
              tunnel: w373 -> [w510 _]
              tunnel: w363 -> [w509 _]
              tunnel: w360 -> [w508 _]
              tunnel: w357 -> [w507 _]
              frame No Error {
                n186 = call "CurrentPlane.vi"("queue In"=w507, "gain"=w509, "bits A/D"=w508, "Axis Vals"=w514, "error in"=w511, "Frame"=w513, "Data"=w510) -> ("error out"=w512:errorcluster, "stop out"=w515:bool)  [unwired: 3 in]
              }
              frame Error {
              }
            }
            n187 = local write "Frames"(w377) -> ()
            n188 = case shown="1, Default" w368 {
              tunnel: w380 -> [_ w388]
              tunnel: w379 -> [_ w387]
              tunnel: w372 -> [_ w386]
              frame 7 {
              }
              frame 1, Default {
                n189 = call <vilib>:"Stop Program.flx"("error in (no error)"=w387, "Program (1)"=w386, "Board ID"=w388) -> ()  [unwired: 6 out]
              }
            }
            n190 = Not(x=w367) -> (.not. x?=w383:bool)
          }
          n191 = global read "MotionGlobals.vi" "motor velocity"() -> (w348)
          n192 = Release Queue(queue=w340) -> ()  [unwired: 2 in, 3 out]
        }
        frame True {
          # "Hack to step through tabor settings."
          n193 = expression code="x*1E-6"(w519) -> (w518:dbl)
          n194 = global read "MotionGlobals.vi" "SavePath"() -> (w527:path)
          n195 = Obtain Queue(max queue size (-1, unlimited)=4, element data type=T8 {"gain"=0.0, TRUE, "Array"=[], "gain 2"=0.0}) -> (queue out=w521:refnum<queue>)  [unwired: 2 in, 3 out]
          n196 = while {
            tunnel: w548 -> [w573]
            tunnel: w521 -> [w572]
            tunnel: [w564] -> w546
            tunnel: w528 -> [w571]
            tunnel: w533 -> [w570]
            tunnel: w534 -> [w569]
            tunnel: w530 -> [w568]
            tunnel: w527 -> [w566]
            tunnel: w526 -> [w565]
            tunnel: w525 -> [w563]
            tunnel: w524 -> [w562]
            tunnel: w523 -> [w561]
            tunnel: w522 -> [w560]
            tunnel: w520 -> [w558]
            tunnel: w518 -> [w557]
            i -> [w574]
            stop <- w564 stop-if-true
            n197 = event shown="[0] Timeout" {
              selector: _ -> [_ _ _ _ _ _ _]
              dyn-events: _ -> [_ _ _ _ _ _ _]
              timeout: 25 -> [_ _ _ _ _ _ _]
              tunnel: w574 -> [w581 _ _ _ _ _ _]
              tunnel: w573 -> [w575 w666 _ _ _ _ _]
              tunnel: [_ _ _ _ _ _ TRUE] -> w564
              tunnel: w572 -> [w585 _ _ _ _ _ _]
              tunnel: w571 -> [_ _ w698 _ _ _ w750]
              tunnel: w570 -> [w584 _ _ _ _ _ w751]
              tunnel: w569 -> [w583 _ _ _ _ _ _]
              tunnel: w568 -> [w582 _ _ _ _ _ _]
              tunnel: "Movie Name" -> [w580 _ _ _ _ _ _]
              tunnel: w566 -> [w579 _ _ _ _ _ _]
              tunnel: w565 -> [w578 _ _ _ _ _ _]
              tunnel: w563 -> [_ _ _ w702 w733 w744 _]
              tunnel: w562 -> [_ _ _ w701 _ _ _]
              tunnel: w561 -> [_ _ _ w700 w735 w746 _]
              tunnel: w560 -> [_ _ _ w699 w734 _ _]
              tunnel: w558 -> [w577 _ _ _ _ _ _]
              tunnel: w557 -> [w576 _ _ _ _ _ _]
              event Timeout {
                n198 = event-data() -> ()  [unwired: 1 in, 2 out]
                n199 = stacked-sequence {
                  tunnel: [w608 _ _] -> _
                  tunnel: w585 -> [w605 _ _]
                  tunnel: w584 -> [w601 _ _]
                  tunnel: w583 -> [w600 _ _]
                  tunnel: w582 -> [w598 _ _]
                  tunnel: w581 -> [w597 w652 _]
                  tunnel: w580 -> [_ w651 _]
                  tunnel: w579 -> [_ w650 _]
                  tunnel: w578 -> [w594 _ _]
                  tunnel: w577 -> [w589 _ _]
                  tunnel: w576 -> [w588 _ _]
                  tunnel: w575 -> [w587 _ _]
                  frame #0 {
                    # "Slightly faster version to read data"
                    # "Get and display data"
                    n200 = Dequeue Element(queue=w605, timeout in ms (-1)=1000) -> (queue out=w608:refnum<queue>, element=w606:T8)  [unwired: 1 in, 2 out]
                    n201 = Unbundle(w606) -> ("gain"=w602:dbl, w603:bool, "Array"=w604:i16[][], "gain 2"=w599:dbl)
                    n202 = case shown="True" w603 {
                      tunnel: w604 -> [w635 w639]
                      tunnel: [w635 w638] -> w596
                      tunnel: w601 -> [_ w637]
                      tunnel: w600 -> [_ w636]
                      frame False {
                      }
                      frame True {
                        n203 = case shown="1" w637 {
                          tunnel: w639 -> [w641 w649]
                          tunnel: [w640 w643] -> w638
                          tunnel: w636 -> [_ w648]
                          frame 0, Default {
                            n204 = call "ReverseData.vi"("Array in"=w641) -> ("Array out"=w640:i16[][])
                          }
                          frame 1 {
                            n205 = Delete From Array(array=w649, length=w648, index (row)=0 ("disabled index (col)")) -> (deleted portion=w646:i16[], array with subset deleted=w647:i16[][])  [unwired: 1 in]
                            n206 = call "ReverseData.vi"("Array in"=w647) -> ("Array out"=w644:i16[][])
                            n207 = call "ReverseData.vi"("Array in"=w646) -> ("Array out"=w645:i16[][])
                            n208 = Build Array (concatenate)(w645, w644) -> (w643:i16[][])
                          }
                        }
                      }
                    }
                    n209 = call "SubMean.vi"("Scan Data In"=w596, "Samp Rate (MHz)"=w588, "Filter Prams"="Filter Prams", "Type of Mean"="Type of Mean") -> ("Array"=w595:dbl[][])  [unwired: 1 out]
                    n210 = case shown="1" "Display mode" {
                      tunnel: [w610 w614 w622 w626 w633] -> w590
                      tunnel: w595 -> [w611 w613 w622 w631 w634]
                      tunnel: w594 -> [_ w612 _ w632 _]
                      tunnel: w589 -> [_ _ _ w625 _]
                      tunnel: w587 -> [_ _ _ w624 _]
                      frame 0, Default {
                        n211 = Absolute Value(x=w611) -> (abs(x)=w610:dbl[][])
                      }
                      frame 1 {
                        n212 = for {
                          tunnel: [w617] -> w614 mode=indexing
                          tunnel: w613 -> [w616] mode=indexing
                          tunnel: w612 -> [w615]
                          n213 = for {
                            tunnel: [w621] -> w617 mode=indexing
                            tunnel: w616 -> [w620] mode=indexing
                            tunnel: w615 -> [w618]
                            n214 = Absolute Value(x=w620) -> (abs(x)=w619:dbl)
                            n215 = Index Array(array=w618, index=w619) -> (element=w621:sgl)
                          }
                        }
                      }
                      frame 2 {
                      }
                      frame 3 {
                        n216 = call "AvisoSectorConvert.vi"("output cluster"=w625, "Log Lookup"=w632, "Raw In"=w631) -> ("Sector out"=w626:dbl[][])  [unwired: 8 in]
                        n217 = Unbundle(w625) -> ("scales"=w627:cluster{"inc x (mm)":dbl, "inc y (mm)":dbl})  [unwired: 4 out]
                        n218 = Unbundle(w627) -> ("inc x (mm)"=w629:dbl, "inc y (mm)"=w628:dbl)
                        n219 = Unbundle(w624) -> (w623:sgl)  [unwired: 4 out]
                        n220 = property on="Raw data" class="IntGraph (strict)"("X Scale.Offset and Multiplier:Offset"=0.0, "X Scale.Offset and Multiplier:Multiplier"=w629, "Y Scale.Offset and Multiplier:Offset"=w623, "Y Scale.Offset and Multiplier:Multiplier"=w628) -> ()  [unwired: 2 in, 2 out]
                      }
                      frame 10 {
                        n221 = expression code="log(abs(x))"(w634) -> (w633:dbl[][])
                      }
                    }
                    "Raw data" <- w590
                    n222 = Increment(x=w597) -> (x+1=w609:i32)
                    "Frames" <- w609
                    n223 = call "SaveEYE_RT_Single.vi"("gain"=w602, 6:w598, "*.eye"="*.eye", "gain 2 Ch"=w599, "Frame"=w609, "Data"=w596) -> ()  [unwired: 6 in]
                  }
                  frame #1 {
                    n224 = case shown="False" "BMP?" {
                      tunnel: w652 -> [_ w656]
                      tunnel: w651 -> [_ w655]
                      tunnel: w650 -> [_ w654]
                      frame False {
                      }
                      frame True {
                        n225 = invoke on="Raw data" class="IntGraph (strict)" method="Get Image"("image depth"=24) -> ("image data"=w657:T16)  [unwired: 5 in, 5 out]
                        n226 = call <vilib>:"Unflatten Pixmap.vi"("image data"=w657) -> ("24-bit pixmap"=w658:u32[][])  [unwired: 10 out]
                        n227 = call "NumberFileName.vi"("String"=".bmp", "File number"=w656, "file name"=w655) -> ("Numbered File"=w662:string)  [unwired: 1 in]
                        n228 = To Unsigned Byte Integer(number=w658) -> (unsigned 8bit integer=w659:u8[][])
                        n229 = call <vilib>:"Flatten Pixmap.vi"("colors"=u32[] [0, 0, 65793, 131586, 197379, 263172, 328965, 394758, 460551, 526344, 592137, 657930, 723723, 789516, 855309, 921102, 986895, 1052688, 1118481, 1184274, 1250067, 1315860, 1381653, 1447446, 1513239, 1579032, 1644825, 1710618, 1776411, 1842204, 1907997, 1973790, 2039583, 2105376, 2171169, 2236962, 2302755, 2368548, 2434341, 2500134, 2565927, 2631720, 2697513, 2763306, 2829099, 2894892, 2960685, 3026478, 3092271, 3158064, 3223857, 3289650, 3355443, 3421236, 3487029, 3552822, 3618615, 3684408, 3750201, 3815994, 3881787, 3947580, 4013373, 4079166, 4144959, 4210752, 4276545, 4342338, 4408131, 4473924, 4539717, 4605510, 4671303, 4737096, 4802889, 4868682, 4934475, 5000268, 5066061, 5131854, 5197647, 5263440, 5329233, 5395026, 5460819, 5526612, 5592405, 5658198, 5723991, 5789784, 5855577, 5921370, 5987163, 6052956, 6118749, 6184542, 6250335, 6316128, 6381921, 6447714, 6513507, 6579300, 6645093, 6710886, 6776679, 6842472, 6908265, 6974058, 7039851, 7105644, 7171437, 7237230, 7303023, 7368816, 7434609, 7500402, 7566195, 7631988, 7697781, 7763574, 7829367, 7895160, 7960953, 8026746, 8092539, 8158332, 8224125, 8289918, 8355711, 8421504, 8487297, 8553090, 8618883, 8684676, 8750469, 8816262, 8882055, 8947848, 9013641, 9079434, 9145227, 9211020, 9276813, 9342606, 9408399, 9474192, 9539985, 9605778, 9671571, 9737364, 9803157, 9868950, 9934743, 10000536, 10066329, 10132122, 10197915, 10263708, 10329501, 10395294, 10461087, 10526880, 10592673, 10658466, 10724259, 10790052, 10855845, 10921638, 10987431, 11053224, 11119017, 11184810, 11250603, 11316396, 11382189, 11447982, 11513775, 11579568, 11645361, 11711154, 11776947, 11842740, 11908533, 11974326, 12040119, 12105912, 12171705, 12237498, 12303291, 12369084, 12434877, 12500670, 12566463, 12632256, 12698049, 12763842, 12829635, 12895428, 12961221, 13027014, 13092807, 13158600, 13224393, 13290186, 13355979, 13421772, 13487565, 13553358, 13619151, 13684944, 13750737, 13816530, 13882323, 13948116, 14013909, 14079702, 14145495, 14211288, 14277081, 14342874, 14408667, 14474460, 14540253, 14606046, 14671839, 14737632, 14803425, 14869218, 14935011, 15000804, 15066597, 15132390, 15198183, 15263976, 15329769, 15395562, 15461355, 15527148, 15592941, 15658734, 15724527, 15790320, 15856113, 15921906, 15987699, 16053492, 16119285, 16185078, 16250871, 16316664, 16382457, 16448250, 16514043, 16579836, 16645629, 16448250] ("Array 2"), "8-bit pixmap"=w659) -> ("image data"=w660:T16)  [unwired: 4 in, 5 out]
                        n230 = Build Path(base path=w654, name or relative path=w662) -> (appended path=w663:path)
                        n231 = call <vilib>:"Write BMP File.vi"("image data"=w660, "path to BMP file"=w663) -> ()  [unwired: 1 in, 9 out]
                      }
                    }
                  }
                  frame #2 {
                  }
                }
              }
              event "distance?", "view": Value Change {
                n232 = event-data() -> ()  [unwired: 1 in, 5 out]
                n233 = case shown="True" "distance?" {
                  tunnel: [w675 w681] -> w673
                  tunnel: [w674 w680] -> w672
                  tunnel: [w675 w679] -> w671
                  tunnel: [w674 w678] -> w670
                  tunnel: "view" -> [_ w683]
                  tunnel: w666 -> [_ w676]
                  frame False {
                    w674 = 1
                    w675 = 0
                  }
                  frame True {
                    n234 = Unbundle(w676) -> (w686:sgl, w685:dbl, w684:dbl, w682:dbl, w677:sgl)
                    n235 = case shown="True" w683 {
                      tunnel: [w690 w694] -> w681
                      tunnel: w686 -> [w690 w691]
                      tunnel: [w689 w693] -> w680
                      tunnel: w685 -> [w689 w692]
                      tunnel: [w688 w691] -> w679
                      tunnel: w684 -> [w688 w694]
                      tunnel: [w687 w692] -> w678
                      tunnel: w682 -> [w687 w693]
                      tunnel: w677 -> [_ _]
                      frame False {
                      }
                      frame True {
                        n236 = Negate(x=w692) -> ()  [unwired: 1 out]
                      }
                    }
                  }
                }
                n237 = Not(x="view") -> (.not. x?=w669:bool)
                n238 = property on="Raw data" class="IntGraph (strict)"("X Scale.Offset and Multiplier:Offset"=w673, "X Scale.Offset and Multiplier:Multiplier"=w672, "Y Scale.Offset and Multiplier:Offset"=w671, "Y Scale.Offset and Multiplier:Multiplier"=w670, "Transpose Array"=w669) -> ()  [unwired: 2 in, 2 out]
              }
              event "Tabor.Tabor Step Through?": Value Change {
                n239 = event-data() -> ()  [unwired: 1 in, 5 out]
                n240 = Enqueue Element(queue=w698, element="Tabor") -> ()  [unwired: 2 in, 3 out]
                n241 = Bundle By Name(cluster="Tabor", "Tabor Step Through?"=FALSE) -> (w696:T2)
                n242 = local write "Tabor"(w696) -> ()
              }
              event "Position (mm) (Abs)": Value Change {
                n243 = event-data() -> ("NewVal"=w703:dbl)  [unwired: 1 in, 4 out]
                n244 = case shown="1, Default" w699 {
                  tunnel: w700 -> [_ w710]
                  tunnel: w701 -> [_ w709]
                  tunnel: w703 -> [_ w707]
                  tunnel: w702 -> [_ w706]
                  frame 0, 7, 8 {
                  }
                  frame 1, Default {
                    n245 = local read "Axis Tune"() -> (w704:enum32{"Axis 1", "Axis 2", "Axis 3", "Axis 4"})
                    n246 = Index Array(array=w706, index=w704) -> (element=w714)
                    n247 = Equal?(x=w704, y=w709) -> (x = y?=w708:bool)
                    n248 = To Byte Integer(number=w704) -> (8bit integer=w711:i8)
                    n249 = Multiply(x=w707, y=w714) -> (x*y=w713:dbl)
                    n250 = Increment(x=w711) -> (x+1=w705:i8)
                    n251 = case shown="\"Axis 3\"" w704 {
                      tunnel: w713 -> [w728 w730]
                      tunnel: [w728 w729] -> w712
                      frame "Axis 1", Default {
                      }
                      frame "Axis 3" {
                        n252 = global read "MotionGlobals.vi" "Reverse Z axis?"() -> (w731)
                        n253 = Negate(x=w730) -> (-x=w732:dbl)
                        n254 = Select(t=w732, s=w731, f=w730) -> (s? t:f=w729:dbl)
                      }
                    }
                    n255 = case shown="True" w708 {
                      tunnel: w705 -> [w723 _]
                      tunnel: w712 -> [w716 _]
                      tunnel: w710 -> [w715 w725]
                      tunnel: w704 -> [_ w726]
                      tunnel: w706 -> [_ w727]
                      frame False {
                        n256 = call <vilib>:"Set Operation Mode.flx"("Axis or Vector Space"=w723, "Board ID"=w715) -> ("error out"=w722:errorcluster, "Resource Output"=w720:T9, "Bd ID Out"=w721:T3)  [unwired: 4 in]
                        n257 = call <vilib>:"Load Target Position.flx"("Target Position (0)"=w716, "error in (no error)"=w722, "Axis"=w720, "Board ID"=w721) -> ("error out"=w718:errorcluster, "Resource Output"=w717:T9, "Bd ID Out"=w719:T3)  [unwired: 3 in]
                        n258 = call-poly <vilib>:"Start Motion.flx"("error in (no error)"=w718, "Axis or Vector Space"=w717, "Board ID"=w719) -> ()  [unwired: 3 in, 3 out]
                      }
                      frame True {
                        n259 = call "FindLocation_SingleAxis.vi"("ct/mm"=w727, "Axis (0 is X)"=w726, "Board ID"=w725) -> ("Position (mm) (Abs)"=w724:dbl)  [unwired: 1 in, 2 out]
                        n260 = local write "Position (mm) (Abs)"(w724) -> ()
                      }
                    }
                  }
                }
              }
              event "Axis Tune": Value Change {
                n261 = event-data() -> ("NewVal"=w736:enum32{"Axis 1", "Axis 2", "Axis 3", "Axis 4"})  [unwired: 1 in]
                n262 = case shown="1, Default" w734 {
                  tunnel: w735 -> [w738 _]
                  tunnel: w733 -> [w740 _]
                  tunnel: w736 -> [w739 _]
                  frame 1, Default {
                    n263 = call "FindLocation_SingleAxis.vi"("ct/mm"=w740, "Axis (0 is X)"=w739, "Board ID"=w738) -> ("Position (mm) (Abs)"=w737:dbl)  [unwired: 1 in, 2 out]
                    n264 = local write "Position (mm) (Abs)"(w737) -> ()
                  }
                  frame 0, 7, 8 {
                  }
                }
              }
              event "Stop Motor": Value Change {
                n265 = event-data() -> ()  [unwired: 1 in, 1 out]
                n266 = local read "Axis Tune"() -> (w743:enum32{"Axis 1", "Axis 2", "Axis 3", "Axis 4"})
                n267 = Increment(x=w743) -> (x+1=w748:enum32{"Axis 1", "Axis 2", "Axis 3", "Axis 4"})
                n268 = call-poly <vilib>:"Stop Motion.flx"("Stop Type (Decel)"=enum16{"Decelerate", "Halt", "Kill"}."Halt", "Axis or Vector Space"=w748, "Board ID"=w746) -> ("error out"=w741:errorcluster, "Bd ID Out"=w745:T3)  [unwired: 4 in, 1 out]
                n269 = call "FindLocation_SingleAxis.vi"("error in (no error)"=w741, "ct/mm"=w744, "Axis (0 is X)"=w743, "Board ID"=w745) -> ("Position (mm) (Abs)"=w742:dbl)  [unwired: 2 out]
                n270 = local write "Position (mm) (Abs)"(w742) -> ()
              }
              event "stop": Value Change {
                n271 = event-data() -> ()  [unwired: 1 in, 2 out]
                n272 = local read "Tabor"() -> (w749:T2)
                n273 = case shown="0, Default" w751 {
                  tunnel: w750 -> [w754 _]
                  tunnel: w749 -> [w753 _]
                  frame 0, Default {
                    n274 = Enqueue Element(queue=w754, element=w753) -> ()  [unwired: 2 in, 3 out]
                  }
                  frame 4, 5 {
                  }
                }
              }
            }
          }
          n275 = while {
            tunnel: w534 -> [w765]
            tunnel: w550 -> [w766]
            tunnel: w523 -> [w767]
            tunnel: w521 -> [w764]
            tunnel: ["stop"] -> w547
            tunnel: w542 -> [w758]
            tunnel: w531 -> [w756]
            stop <- "stop" stop-if-true
            # "Slightly faster version to read data"
            # "Get and display data"
            n276 = call "Rapid Read.vi"("Channel"=w756, "lines per plane"=w765, "rf points per line"=w766, "Motion Board ID"=w767, "NI Card"=w758) -> ("Reverse?"=w762:bool, "Array"=w761:i16[][], "gain 2 Ch"=w757:dbl, "gain"=w759:dbl)  [unwired: 1 in, 2 out]
            n277 = Not(x=w762) -> (.not. x?=w755:bool)
            n278 = Bundle("gain"=w759, w755, "Array"=w761, "gain 2 Ch"=w757) -> (w760:T17)  [unwired: 1 out]
            n279 = Lossy Enqueue Element(queue=w764, element=w760) -> ()  [unwired: 1 in, 4 out]
          }
          n280 = And(x=w547, y=w546) -> (x .and. y?=w545:bool)
          n281 = Release Queue(queue=w521, force destroy? (F)=w545) -> (error out=w536:errorcluster)  [unwired: 1 in, 2 out]
          n282 = Dequeue Element(queue=w528) -> (element=w541:T2, error out=w532:errorcluster)  [unwired: 2 in, 2 out]
          n283 = Lossy Enqueue Element(queue=w528, element=w529, error in (no error)=w536) -> (queue out=w535:refnum<queue>)  [unwired: 3 out]
          n284 = Unbundle(w541) -> ("Time Step (ms)"=w539:i64, "Burst Ct"=w538:i8[], "Voltage Steps"=w537:sgl[], "Tabor Step Through?"=w540:bool)
          n285 = Release Queue(queue=w535, error in (no error)=w532) -> ()  [unwired: 1 in, 3 out]
          n286 = case shown="False" w540 {
            tunnel: w539 -> [_ w553]
            tunnel: w538 -> [_ w552]
            tunnel: w537 -> [_ w551]
            frame False {
            }
            frame True {
              n287 = flat-sequence {
                tunnel: w553 -> [w556]
                tunnel: w552 -> [w555]
                tunnel: w551 -> [w554]
                frame #0 {
                  n288 = call "TaborSkipThrough.vi"("Voltage Steps"=w554, "Burst Ct"=w555, "Time Step (ms)"=w556) -> ()  [unwired: 9 in]
                }
                frame #1 {
                  n289 = call <vilib>:"Beep.vi"() -> ()  [unwired: 12 in]
                }
              }
            }
          }
        }
      }
    }
    frame #6 {
      n290 = case shown="\"Hawaii\", Default" w775 {
        frame "Hawaii", Default {
          # "turn off real time trig"
          n291 = call-poly <vilib>:"DAQmx Write.vi"("task/channels in"=refnum<k21> "DIO-L2 L3", "data"=bool[] [TRUE, FALSE]) -> ()  [unwired: 11 in, 3 out]
        }
        frame "UHI Allen", "CUMC RT" {
        }
      }
      n292 = case shown="4, 5" w773 {
        tunnel: w772 -> [_ w776]
        frame 0, Default {
        }
        frame 4, 5 {
          n293 = for {
            tunnel: w776 -> [w779] mode=indexing
            n294 = call <vilib>:"DAQmx Stop Task.vi"("task/channels in"=w779) -> ("task out"=w778:refnum<k21>, "error out"=w777:errorcluster)  [unwired: 13 in]
            n295 = call <vilib>:"DAQmx Clear Task.vi"("task in"=w778, "error in"=w777) -> ()  [unwired: 13 in, 1 out]
          }
        }
      }
      n296 = local read "Movie Name"() -> (w768:string)
      n297 = Concatenate Strings(w768, "a" ("string")) -> (w770:string)
      n298 = local write "Movie Name"(w770) -> ()
      n299 = local write "BMP?"(FALSE) -> ()
      n300 = local write "stop"(FALSE ("stop out")) -> ()
    }
  }
  n301 = case shown="1, Default" w20 {
    tunnel: w37 -> [w787 w803 _]
    tunnel: w36 -> [_ w802 _]
    tunnel: w35 -> [_ w801 _]
    tunnel: w34 -> [w783 w800 w829]
    tunnel: w33 -> [w786 w799 _]
    tunnel: w31 -> [_ w795 _]
    tunnel: w24 -> [w785 w794 _]
    tunnel: w23 -> [_ w793 _]
    tunnel: w19 -> [w784 _ _]
    tunnel: [w782 w792 w829] -> w18
    frame 7 {
      n302 = call <instrlib>:"Move Absolute.vi"("error in (no error)"=w783, "Position (0 units)"=w786, "Axis (1)"=w787, "VISA resource name"=w784) -> ("error out"=w790:errorcluster, "VISA resource name out"=w788:refnum<visa-resource-name>)  [unwired: 2 in]
      n303 = call <instrlib>:"Set Velocity.vi"("error in (no error)"=w790, "Velocity (units/s)"=w785, "Axis (1)"=w787, "VISA resource name"=w788) -> ("error out"=w782:errorcluster, "VISA resource name out"=w789:refnum<visa-resource-name>)  [unwired: 2 in]
      n304 = call "WaitStopEPS.vi"("VISA resource name"=w789) -> ()  [unwired: 2 in, 3 out]
    }
    frame 1, Default {
      n305 = case shown="True" w795 {
        tunnel: w802 -> [w823 w828]
        tunnel: w801 -> [_ w827]
        tunnel: w800 -> [w822 w826]
        tunnel: [w823 w825] -> w798
        tunnel: [w822 w824] -> w797
        frame False {
        }
        frame True {
          n306 = call <vilib>:"Stop Program.flx"("error in (no error)"=w826, "Program (1)"=w827, "Board ID"=w828) -> ("error out"=w824:errorcluster, "Bd ID Out"=w825:T3)  [unwired: 4 out]
        }
      }
      n307 = case shown="True" "return to start" {
        tunnel: w803 -> [_ w811]
        tunnel: w799 -> [_ w819]
        tunnel: w798 -> [w805 w810]
        tunnel: w797 -> [w804 w809]
        tunnel: [w805 w818] -> w796
        tunnel: w794 -> [_ w817]
        tunnel: w793 -> [_ w816]
        tunnel: [w804 w815] -> w792
        frame False {
        }
        frame True {
          n308 = call "MoveMotor.vi"("error in (no error)"=w809, "Target Position (0)"=w819, "Axis or Vector Space"=w811, "Motion Bd ID"=w810) -> ("error out"=w807:errorcluster, "Resource Output"=w806:u16, "Bd ID Out"=w808:u8)  [unwired: 1 in, 4 out]
          n309 = call "Load Acceleration/Deceleration.flx"("Acceleration (100000)"=w816, "error in (no error)"=w807, "Axis or Vector Space"=w806, "Board ID"=w808) -> ("error out"=w814:errorcluster, "Resource Output"=w812:T9, "Bd ID Out"=w813:T3)  [unwired: 1 in, 2 out]
          n310 = call <vilib>:"Load Velocity.flx"("Velocity (10000)"=w817, "error in (no error)"=w814, "Axis or Vector Space"=w812, "Board ID"=w813) -> ("error out"=w815:errorcluster, "Bd ID Out"=w818:T3)  [unwired: 4 out]
        }
      }
      n311 = flat-sequence {
        tunnel: w796 -> [w820]
        frame #0 {
          "Bd ID Out" <- w820
        }
        frame #1 {
          n312 = Wait (ms)(milliseconds to wait=u32 10) -> ()  [unwired: 1 out]
        }
      }
    }
    frame 8 {
    }
  }
  "error out" <- w18
